vi "memory_stub.vi"() -> ()   [LabVIEW 2024, in "Nominal Client Engine.lvlib"]
uses:
  <vilib>/LabVIEW Open Source Project/Epoch Date & Time/formatter.iso8601/DateTime.ISO8601.lvclass
  <vilib>/LabVIEW Open Source Project/Epoch Date & Time/formatter.iso8601/ISO8601 Date Formats.ctl
  <vilib>/LabVIEW Open Source Project/Epoch Date & Time/formatter/DateTimeFormatter.lvclass
  <vilib>/LabVIEW Open Source Project/Epoch Date & Time/epoch.GPS/Epoch.GPS.lvclass
  <vilib>/LabVIEW Open Source Project/Epoch Date & Time/epoch/Epoch.lvclass
  <vilib>/LabVIEW Open Source Project/Epoch Date & Time/epoch.UNIX/Epoch.UNIX.lvclass
  <vilib>/LabVIEW Open Source Project/Epoch Date & Time/epoch.UTC/Epoch.UTC.lvclass
  <vilib>/LabVIEW Open Source Project/Epoch Date & Time/Epochs -- enum.ctl
  <vilib>/LabVIEW Open Source Project/Epoch Date & Time/UTC Offsets -- enum.ctl
  <vilib>/Nominal/Nominal IO Client/Nominal Client MultiPart Upload/Multipart Upload.lvclass
  <vilib>/Nominal/Nominal IO Client/Nominal Client/Nominal Client.lvclass
  <vilib>/addons/_JKI.lib/REST Client/classes/REST Client/REST Client.lvclass
  <vilib>/Utility/lvfile.llb/FT_FileTypes.ctl
  <vilib>/picture/picture.llb/imagedata.ctl
  <vilib>/addons/_JKI.lib/REST Client/classes/Response Headers/Response Headers.lvclass
  <vilib>/addons/_JKI.lib/REST Client/classes/REST Client/HTTP Header.ctl
  <vilib>/NI/Advanced HTTP Client/Header--Combo Box.ctl
  <vilib>/httpClient/MultipartData.ctl
  <vilib>/Nominal/Nominal IO Client/Run/Run.lvclass
  <vilib>/Nominal/Nominal IO Client/Run/Run Data.ctl
  <vilib>/LabVIEW Open Source Project/Epoch Date & Time/formatter.iso8601/ISO Day -- enum.ctl
  <vilib>/Nominal/Nominal IO Client/timestampMetadata/timestampMetadata.lvclass
  <vilib>/Utility/error.llb/whitespace.ctl
  <vilib>/Nominal/Nominal IO Client/ts.epochOfTimeUnit/ts.epochOfTimeUnit.lvclass
  <vilib>/Nominal/Nominal IO Client/ts.iso8601/ts.iso8601.lvclass
  <vilib>/Nominal/Nominal IO Client/ts.relative/ts.relative.lvclass
  Engine/Nominal Client Engine.lvlib
  <userlib>/_OpenG.lib/array/array.llb/openg_array.lvlib
  <userlib>/_OpenG.lib/array/array.llb/Conditional Auto-Indexing Tunnel (DBL)__ogtk.vi
  <userlib>/_OpenG.lib/array/array.llb/Delete Elements from 1D Array (DBL)__ogtk.vi
  <userlib>/_OpenG.lib/array/array.llb/Empty 1D Array (DBL)__ogtk.vi
  <userlib>/_OpenG.lib/array/array.llb/Filter 1D Array (DBL)__ogtk.vi
  <userlib>/_OpenG.lib/array/array.llb/Index 1D Array Elements (DBL)__ogtk.vi
  <userlib>/_OpenG.lib/array/array.llb/Remove Duplicates from 1D Array (DBL)__ogtk.vi
  <userlib>/_OpenG.lib/array/array.llb/Reorder 1D Array2 (DBL)__ogtk.vi
  <userlib>/_OpenG.lib/array/array.llb/Reorder 1D Array (DBL)__ogtk.vi
  <userlib>/_OpenG.lib/array/array.llb/Reverse 2D Array (Variant)__ogtk.vi
  <userlib>/_OpenG.lib/array/array.llb/Search 1D Array (DBL)__ogtk.vi
  <userlib>/_OpenG.lib/array/array.llb/Slice 1D Array (DBL)__ogtk.vi
  <userlib>/_OpenG.lib/array/array.llb/Sort 2D Array (DBL)__ogtk.vi
  <userlib>/_OpenG.lib/array/array.llb/Sort 1D Array (DBL)__ogtk.vi
  <vilib>/JDP Science/JDP Science Common Utilities/Base64/Base64 Support.lvlib
  <vilib>/Utility/Data Type/NI_Data Type.lvlib
  <vilib>/Utility/lvfile.llb/NI_FileType.lvlib
  <vilib>/Utility/LVLibp/NI_PackedLibraryUtility.lvlib
  <vilib>/NI/Advanced HTTP Client/Session.lvclass
  <vilib>/httpClient/LabVIEWHTTPClient.lvlib
panel:
  in  "prompt":string
  in  "error in":errorcluster
  in  "append to file? (new file:F)":bool
  in  "spreadsheet string":string
  in  "file path (dialog if empty)":path
  out "error out":errorcluster
  out "path":path
  in  "file path (dialog if empty) 2":path
  in  "format (%.3f)":string="%.3f"
  in  "2D data":dbl[][](array[numeric])
  in  "1D data":dbl[](array[numeric])
  in  "append to file? (new file:F) 2":bool
  in  "error in (no error)":errorcluster
  in  "transpose? (no:F)":bool
  in  "delimiter (\\t)":string="\t"
  out "new file path (Not A Path if cancelled)":path
  out "error out 2":errorcluster
  in  "file path (dialog if empty) 3":path
  in  "format (%s)":string="%s"
  in  "2D data 2":string[][](array[string])
  in  "1D data 2":string[](array[string])
  in  "append to file? (new file:F) 3":bool
  in  "error in (no error) 2":errorcluster
  in  "transpose? (no:F) 2":bool
  in  "delimiter (\\t) 2":string="\t"
  out "new file path (Not A Path if cancelled) 2":path
  out "error out 3":errorcluster
  in  "file path (dialog if empty) 4":path
  in  "format (%d)":string="%d"
  in  "2D data 3":i64[][](array[numeric])
  in  "1D data 3":i64[](array[numeric])
  in  "append to file? (new file:F) 4":bool
  in  "error in (no error) 3":errorcluster
  in  "transpose? (no:F) 3":bool
  in  "delimiter (\\t) 3":string="\t"
  out "new file path (Not A Path if cancelled) 3":path
  out "error out 4":errorcluster
  in  "file path (dialog if empty) 5":path
  in  "format (%.3f) 2":string="%.3f"
  in  "2D data 4":dbl[][](array[numeric])
  in  "1D data 4":dbl[](array[numeric])
  in  "append to file? (new file:F) 5":bool
  in  "error in (no error) 4":errorcluster
  in  "transpose? (no:F) 4":bool
  in  "delimiter (\\t) 4":string="\t"
  out "new file path (Not A Path if cancelled) 4":path
  out "error out 5":errorcluster
  in  "UTC Offset String":string
  out "Valid?":bool
  out "Offset (s)":ext
  out "UTC Offset":T1=enum."UTC+00:00"
  out "UTC Offset?":bool
  in  "error in 2":errorcluster
  in  "ts.relative in":refnum<class "ts.relative.lvclass">
  out "error out 6":errorcluster
  out "JSON Object":string
  out "ts.relative out":refnum<class "ts.relative.lvclass">
  in  "Time Unit":T2(ring)
  in  "Time Series Name":string
  out "ts.relative out 2":refnum<class "ts.relative.lvclass">
  in  "error in 3":errorcluster
  in  "ts.iso8601 in":refnum<class "ts.iso8601.lvclass">
  out "error out 7":errorcluster
  out "JSON Object 2":string
  out "ts.iso8601 out":refnum<class "ts.iso8601.lvclass">
  in  "Time Series Name 2":string
  out "ts.iso8601 out 2":refnum<class "ts.iso8601.lvclass">
  in  "error in 4":errorcluster
  in  "ts.epochOfTimeUnit in":refnum<class "ts.epochOfTimeUnit.lvclass">
  out "error out 8":errorcluster
  out "JSON Object 3":string
  out "ts.epochOfTimeUnit out":refnum<class "ts.epochOfTimeUnit.lvclass">
  in  "Time Unit 2":T2(ring)
  in  "Time Series Name 3":string
  out "ts.epochOfTimeUnit out 2":refnum<class "ts.epochOfTimeUnit.lvclass">
  in  "string":string
  in  "location (both)":T3 items=["both", "start of string", "end of string"]
  out "trimmed string":string
  in  "string 2":string
  in  "reverse?":bool
  in  "enable?":bool
  out "trimmed string 2":string
  out "timestampMetadata out":refnum<class "timestampMetadata.lvclass">
  in  "error in 5":errorcluster
  in  "Object To Update":string
  in  "JSON in":string
  in  "timestampMetadata in":refnum<class "timestampMetadata.lvclass">
  out "error out 9":errorcluster
  out "JSON out":string
  out "timestampMetadata out 2":refnum<class "timestampMetadata.lvclass">
  in  "error in 6":errorcluster
  in  "Object Name":string="timestampMetadata"
  in  "JSON in 2":string
  in  "timestampMetadata in 2":refnum<class "timestampMetadata.lvclass">
  out "error out 10":errorcluster
  out "JSON out 2":string
  out "timestampMetadata out 3":refnum<class "timestampMetadata.lvclass">
  in  "error in 7":errorcluster
  in  "timestampMetadata in 3":refnum<class "timestampMetadata.lvclass">
  out "error out 11":errorcluster
  out "JSON Object 4":string
  out "timestampMetadata out 4":refnum<class "timestampMetadata.lvclass">
  out "timestampMetadata out 5":refnum<class "timestampMetadata.lvclass">
  in  "UTC? (F)":bool
  in  "Timestamp (now)":timestamp
  out "is Leap Year?":bool
  out "year":i32
  in  "UTC? (F) 2":bool
  in  "Timestamp (now) 2":timestamp
  out "ISO8601 Ordinal Date":string
  out "ISO8601 Weekday":string
  out "ISO8601 Week":string
  in  "UTC? (F) 3":bool
  in  "Timestamp (now) 3":timestamp
  out "ISO8601 UTC DateTime":string
  in  "UTC? (F) 4":bool
  in  "Timestamp (now) 4":timestamp
  out "Day of Year":i32
  out "ISO Weekday":i32
  out "ISO Day":T4
  in  "UTC? (F) 5":bool
  in  "Timestamp (now) 5":timestamp
  out "ISO8601 Calendar Month":string
  out "ISO8601 Date":string
  out "String":string
  in  "Run Data":T5
  out "Run":refnum<class "Run.lvclass">
  in  "error in (no error) 5":errorcluster
  in  "REST Client in":refnum<class "REST Client.lvclass">
  out "error out 12":errorcluster
  in  "request specific headers":T6[](array[typedef])
  in  "timeout (0 = Use Default)":i32
  in  "error in (no error) 6":errorcluster
  in  "Request body":string
  in  "Path":string
  in  "REST Client in 2":refnum<class "REST Client.lvclass">
  out "error out 13":errorcluster
  out "Response body":string
  out "Response Headers":refnum<class "Response Headers.lvclass">
  out "REST Client out":refnum<class "REST Client.lvclass">
  out "Status String":string
  out "Status Code":u16
  in  "request specific headers 2":T6[](array[typedef])
  in  "timeout (0 = Use Default) 2":i32
  in  "error in (no error) 7":errorcluster
  in  "Path 2":string
  in  "REST Client in 3":refnum<class "REST Client.lvclass">
  out "error out 14":errorcluster
  out "Response body 2":string
  out "Response Headers 2":refnum<class "Response Headers.lvclass">
  out "REST Client out 2":refnum<class "REST Client.lvclass">
  out "Status String 2":string
  out "Status Code 2":u16
  in  "request specific headers 3":T6[](array[typedef])
  in  "timeout (0 = Use Default) 3":i32
  in  "error in (no error) 8":errorcluster
  in  "Multipart Post data":T8[](array[typedef])
  in  "Path 3":string
  in  "REST Client in 4":refnum<class "REST Client.lvclass">
  out "error out 15":errorcluster
  out "Response body 3":string
  out "Response Headers 3":refnum<class "Response Headers.lvclass">
  out "REST Client out 3":refnum<class "REST Client.lvclass">
  out "Status String 3":string
  out "Status Code 3":u16
  in  "request specific headers 4":T6[](array[typedef])
  in  "timeout (0 = Use Default) 4":i32
  in  "error in (no error) 9":errorcluster
  in  "Request body 2":string
  in  "Path 4":string
  in  "REST Client in 5":refnum<class "REST Client.lvclass">
  out "error out 16":errorcluster
  out "Response body 4":string
  out "Response Headers 4":refnum<class "Response Headers.lvclass">
  out "REST Client out 4":refnum<class "REST Client.lvclass">
  out "Status String 4":string
  out "Status Code 4":u16
  in  "request specific headers 5":T6[](array[typedef])
  in  "timeout (0 = Use Default) 5":i32
  in  "error in (no error) 10":errorcluster
  in  "Request body 3":string
  in  "Path 5":string
  in  "REST Client in 6":refnum<class "REST Client.lvclass">
  out "error out 17":errorcluster
  out "Response body 5":string
  out "Response Headers 5":refnum<class "Response Headers.lvclass">
  out "REST Client out 5":refnum<class "REST Client.lvclass">
  out "Status String 5":string
  out "Status Code 5":u16
  in  "request specific headers 6":T6[](array[typedef])
  in  "timeout (0 = Use Default) 6":i32
  in  "error in (no error) 11":errorcluster
  in  "Path 6":string
  in  "REST Client in 7":refnum<class "REST Client.lvclass">
  out "error out 18":errorcluster
  out "Response body 6":string
  out "Response Headers 6":refnum<class "Response Headers.lvclass">
  out "REST Client out 6":refnum<class "REST Client.lvclass">
  out "Status String 6":string
  out "Status Code 6":u16
  in  "request specific headers 7":T6[](array[typedef])
  in  "timeout (0 = Use Default) 7":i32
  in  "error in (no error) 12":errorcluster
  in  "Path 7":string
  in  "REST Client in 8":refnum<class "REST Client.lvclass">
  out "error out 19":errorcluster
  out "Response body 7":string
  out "Response Headers 7":refnum<class "Response Headers.lvclass">
  out "REST Client out 7":refnum<class "REST Client.lvclass">
  out "Status String 7":string
  out "Status Code 7":u16
  in  "Default Headers ([JSON])":T6[](array[typedef])=[{"header"="Content-Type", "value"="application/json"}]
  in  "REST Client in 9":refnum<class "REST Client.lvclass">
  in  "Verify Server(true)":bool=TRUE
  in  "Cookie File":path
  in  "error in (no error) 13":errorcluster
  in  "Authentication":cluster{"Username":string, "Password":string}
  in  "Escape URLs (true)":bool=TRUE
  in  "Base URL":string
  out "error out 20":errorcluster
  out "REST Client out 8":refnum<class "REST Client.lvclass">
  in  "error in (no error) 14":errorcluster
  in  "Response Headers in":refnum<class "Response Headers.lvclass">
  out "error out 21":errorcluster
  out "Values":string[](array[string])
  out "Names":string[](array[string])
  out "Response Headers out":refnum<class "Response Headers.lvclass">
  in  "error in (no error) 15":errorcluster
  in  "Name":string
  in  "Response Headers in 2":refnum<class "Response Headers.lvclass">
  out "error out 22":errorcluster
  out "Found?":bool
  out "Value":string
  out "Response Headers out 2":refnum<class "Response Headers.lvclass">
  in  "error in (no error) 16":errorcluster
  in  "vi reference":refnum<vi>
  out "error out 25":errorcluster
  out "packed library path":path
  out "vi reference out":refnum<vi>
  in  "error in (no error) 17":errorcluster
  in  "packed library path 2":path
  out "error out 26":errorcluster
  out "source project path":path
  in  "error in (no error) 18":errorcluster
  in  "packed library path 3":path
  out "error out 27":errorcluster
  out "guid":string
  in  "error in (no error) 19":errorcluster
  in  "qualified name":string
  in  "packed library path 4":path
  out "error out 28":errorcluster
  out "path 2":path
  in  "error in (no error) 20":errorcluster
  in  "packed library path 5":path
  out "error out 29":errorcluster
  out "paths":path[](array[path])
  out "qualified names":string[](array[string])
  in  "error in (no error) 21":errorcluster
  in  "Enable":bool
  out "error out 30":errorcluster
  in  "file type":T9
  out "Is LabVIEW document?":bool
  in  "file type 2":T9
  out "Is library type?":bool
  in  "file type 3":T9
  out "Can be in LLB?":bool
  in  "error in (no error) 22":errorcluster
  in  "is template?":bool
  in  "file type 4":T9
  out "error out 31":errorcluster
  out "image data":T10
  in  "file type 5":T9
  out "Is VI?":bool
  in  "error in (no error) 23":errorcluster
  in  "path 3":path
  out "error out 32":errorcluster
  out "Is LLB?":bool
  in  "error in (no error) 24":errorcluster
  in  "path 4":path
  out "error out 33":errorcluster
  out "Is Class Private Data Control?":bool
  out "Is VI? 2":bool
  in  "error in (no error) 25":errorcluster
  in  "path 5":path
  out "error out 34":errorcluster
  out "Is library type? 2":bool
  in  "error in (no error) 26":errorcluster
  in  "path 6":path
  out "error out 35":errorcluster
  out "Is LabVIEW document? 2":bool
  in  "error in (no error) 27":errorcluster
  in  "path 7":path
  out "error out 36":errorcluster
  out "image data 2":T10
  in  "error in (no error) 28":errorcluster
  in  "path 8":path
  out "error out 37":errorcluster
  out "is template? 2":bool
  out "file type 6":T9
  in  "error in (no error) 29":errorcluster
  in  "path 9":path
  out "error out 38":errorcluster
  out "Can be in LLB? 2":bool
  in  "error in (no error) 30":errorcluster
  in  "variant":variant
  out "error out 39":errorcluster
  out "default palette path":path
  in  "error in 10":errorcluster
  in  "Multipart Upload in":refnum<class "Multipart Upload.lvclass">
  out "error out 40":errorcluster
  out "Multipart Upload out":refnum<class "Multipart Upload.lvclass">
  in  "Part Number":i32
  in  "error in 11":errorcluster
  in  "File Part Binary":string
  in  "Multipart Upload":refnum<class "Multipart Upload.lvclass">
  out "error out 41":errorcluster
  out "Multipart Upload out 2":refnum<class "Multipart Upload.lvclass">
  in  "Part Number 2":i32
  in  "error in 12":errorcluster
  in  "Multipart Upload in 2":refnum<class "Multipart Upload.lvclass">
  out "error out 42":errorcluster
  out "Multipart Upload out 3":refnum<class "Multipart Upload.lvclass">
  in  "error in 13":errorcluster
  in  "Body":string
  in  "Full Path":string
  in  "REST Client":refnum<class "REST Client.lvclass">
  out "error out 43":errorcluster
  out "Response":string
  in  "error in 14":errorcluster
  in  "Multipart Upload 2":refnum<class "Multipart Upload.lvclass">
  out "error out 44":errorcluster
  out "Multipart Upload out 4":refnum<class "Multipart Upload.lvclass">
  in  "error in 15":errorcluster
  in  "File Path":path
  in  "Nominal Client in":refnum<class "Nominal Client.lvclass">
  out "error out 45":errorcluster
  out "Multipart Upload 3":refnum<class "Multipart Upload.lvclass">
  out "Nominal Client out":refnum<class "Nominal Client.lvclass">
  in  "error in 16":errorcluster
  in  "Multipart Upload in 3":refnum<class "Multipart Upload.lvclass">
  out "error out 46":errorcluster
  out "S3 Path to File":string
  in  "error in 17":errorcluster
  in  "Multipart Upload 4":refnum<class "Multipart Upload.lvclass">
  out "error out 47":errorcluster
  in  "error in 18":errorcluster
  in  "MultiPart Upload":refnum<class "Multipart Upload.lvclass">
  out "error out 48":errorcluster
  in  "error in 19":errorcluster
  in  "Key":string
  in  "Upload ID":string
  out "error out 49":errorcluster
  out "Nominal Client MultiPart Upload":refnum<class "Multipart Upload.lvclass">
  in  "Adjust for Local DST? (T)":bool=TRUE
  in  "Strict ISO? (T)":bool=TRUE
  in  "ISO8601 Date String":string
  out "valid?":bool
  out "ISO Format":T11
  out "Timestamp":timestamp
  in  "timestamp (now)":timestamp
  out "is Leap Year? 2":bool
  in  "Year (0: this year)":i32
  out "is Leap Year? 3":bool
  in  "timestamp (now) 2":timestamp
  out "is DST?":bool
  in  "path 10":path
  out "Is Path and Not Empty?":bool
  in  "Year (0: this year) 2":i32
  out "Month Lengths":i32[](array[numeric])
  in  "error in (no error) 31":errorcluster
  in  "object":refnum<class>
  out "error out 50":errorcluster
  out "class name":string
  in  "UTC? (F) 6":bool
  out "UTC Offset String 2":string
  out "UTC Offset 2":T1=enum."UTC+00:00"
  in  "error in (no error) 32":errorcluster
  in  "file":path
  out "error out 51":errorcluster
  out "filename without extension":string
  out "lowercase file extension":string
  out "dup file":path
  out "unmodified file extension":string
  in  "Timestamp (now) 6":timestamp
  in  "Epoch (Local)":refnum<class "Epoch.lvclass">
  out "Fractional Second":dbl format="%#.19f"
  out "Epoch Time (s)":i64
  out "Epoch out":refnum<class "Epoch.lvclass">
  in  "is warning? (False)":bool
  in  "show call chain? (False)":bool
  in  "error in (no error) 33":errorcluster
  in  "error message (\"\")":string
  in  "error code (0)":i32
  out "error out 52":errorcluster
  in  "Epoch (UTC)":T12=enum."UTC"
  in  "Epoch Time":ext format="%#.6f"
  out "Not a Timestamp?":bool
  in  "Use TAI Offset?":bool
  in  "Fractional Second 2":dbl format="%#.6f"
  in  "UTC Time (s)":i64
  in  "Epoch (UTC) 2":refnum<class "Epoch.UTC.lvclass">
  out "Not a Timestamp? 2":bool
  out "Timestamp 2":timestamp
  out "Epoch out 2":refnum<class "Epoch.UTC.lvclass">
  in  "Epoch":refnum<class "Epoch.UTC.lvclass">
  out "Offset to UTC":i64
  in  "Use TAI Offset? 2":bool
  in  "Fractional Second 3":dbl format="%#.6f"
  in  "Unix Time (s)":i64
  in  "Epoch (Unix)":refnum<class "Epoch.UNIX.lvclass">
  out "Not a Timestamp? 3":bool
  out "Timestamp 3":timestamp
  out "Epoch out 3":refnum<class "Epoch.UNIX.lvclass">
  in  "Epoch (UNIX)":refnum<class "Epoch.UNIX.lvclass">
  out "Offset to UTC 2":i64
  in  "(Integer) Time (us)":i64
  in  "Epoch in":refnum<class "Epoch.lvclass">
  out "Fractional Second 4":dbl format="%#.6f"
  out "(Integer) Time (s)":i64
  out "Epoch out 4":refnum<class "Epoch.lvclass">
  in  "(Integer) Time (ms)":i64
  in  "Epoch in 2":refnum<class "Epoch.lvclass">
  out "Fractional Second 5":dbl format="%#.6f"
  out "(Integer) Time (s) 2":i64
  out "Epoch out 5":refnum<class "Epoch.lvclass">
  in  "(Float) Time (s)":dbl format="%#.6f"
  in  "Epoch in 3":refnum<class "Epoch.lvclass">
  out "Fractional Second 6":dbl format="%#.6f"
  out "(Integer) Time (s) 3":i64
  out "Epoch out 6":refnum<class "Epoch.lvclass">
  in  "Fractional Second 7":dbl format="%#.6f"
  in  "(Integer) Time (s) 4":i64
  in  "Epoch in 4":refnum<class "Epoch.lvclass">
  out "(Integer) Time (us) 2":i64
  out "Epoch out 7":refnum<class "Epoch.lvclass">
  in  "Fractional Second 8":dbl format="%#.6f"
  in  "(Integer) Time (s) 5":i64
  in  "Epoch in 5":refnum<class "Epoch.lvclass">
  out "(Integer) Time (ms) 2":i64
  out "Epoch out 8":refnum<class "Epoch.lvclass">
  in  "Fractional Second 9":dbl format="%#.6f"
  in  "(Integer) Time (s) 6":i64
  in  "Epoch in 6":refnum<class "Epoch.lvclass">
  out "(Float) Time (s) 2":dbl format="%#.6f"
  out "Epoch out 9":refnum<class "Epoch.lvclass">
  in  "UTC Epoch Time":i64=2272060800
  out "Leap Seconds":i64=2272060800
  out "Leap Seconds 2":i64[](array[numeric])
  out "UTC Time":i64[](array[numeric])
  in  "DateTimeFormatter (ISO8601)":refnum<class "DateTimeFormatter.lvclass">
  in  "UTC? (F) 7":bool
  in  "Fractional Second 10":dbl format="%#.6f"
  in  "Epoch Time (s) 2":i64
  in  "Epoch 2":refnum<class "Epoch.lvclass">
  out "Not a Timestamp? 4":bool
  out "DateTime string":string
  out "Epoch out 10":refnum<class "Epoch.lvclass">
  in  "Use TAI Offset? 3":bool
  in  "Fractional Second 11":dbl format="%#.6f"
  in  "Epoch Time (s) 3":i64
  in  "Epoch (Local) 2":refnum<class "Epoch.lvclass">
  out "Not a Timestamp? 5":bool
  out "Timestamp 4":timestamp
  out "Epoch (out)":refnum<class "Epoch.lvclass">
  in  "Reference Time":timestamp
  out "Timestamp Offset":i64
  in  "Epoch Time 2":i64=2272060800
  in  "Epoch 3":refnum<class "Epoch.lvclass">
  out "Offset to TAI":i64
  in  "Epoch 4":refnum<class "Epoch.lvclass">
  out "Offset to UTC 3":i64
  in  "Use TAI Offset? 4":bool=TRUE
  in  "Fractional Second 12":dbl format="%#.6f"
  in  "GPS Time (s)":i64
  in  "Epoch (GPS)":refnum<class "Epoch.GPS.lvclass">
  out "Not a Timestamp? 6":bool
  out "Timestamp 5":timestamp
  out "Epoch out 11":refnum<class "Epoch.GPS.lvclass">
  in  "Epoch (GPS) 2":refnum<class "Epoch.GPS.lvclass">
  out "Offset to UTC 4":i64
  in  "Epoch Time 3":i64=2272060800
  in  "Epoch.GPS":refnum<class "Epoch.GPS.lvclass">
  out "Offset to TAI 2":i64
  in  "DateTime String":string
  in  "DateTimeFormatter in":refnum<class "DateTimeFormatter.lvclass">
  out "Timestamp 6":timestamp
  out "DateTimeFormatter out":refnum<class "DateTimeFormatter.lvclass">
  in  "UTC? (F) 8":bool
  in  "Timestamp (now) 7":timestamp
  in  "DateTimeFormatter in 2":refnum<class "DateTimeFormatter.lvclass">
  out "DateTime String 2":string
  out "DateTimeFormatter out 2":refnum<class "DateTimeFormatter.lvclass">
  in  "DateTime String 3":string
  in  "DateTimeFormatter in 3":refnum<class "DateTimeFormatter.lvclass">
  out "Not a Timestamp? 7":bool
  out "Timestamp 7":timestamp
  out "DateTimeFormatter out 3":refnum<class "DateTimeFormatter.lvclass">
  in  "UTC? (F) 9":bool
  in  "Timestamp (now) 8":timestamp
  in  "DateTimeFormatter in 4":refnum<class "DateTimeFormatter.lvclass">
  out "Not a Timestamp? 8":bool
  out "DateTime String 4":string
  out "DateTimeFormatter out 4":refnum<class "DateTimeFormatter.lvclass">
  in  "Adjust for DST? (T)":bool=TRUE
  in  "Timestamp 8":timestamp
  out "Adjusted Timestamp":timestamp
  in  "year 2":i32
  out "First Day of W01":timestamp
  in  "DateTime String 5":string
  in  "DateTime.ISO8601 in":refnum<class "DateTime.ISO8601.lvclass">
  out "Timestamp 9":timestamp
  out "DateTime.ISO8601 out":refnum<class "DateTime.ISO8601.lvclass">
  in  "UTC? (F) 10":bool
  in  "Timestamp (now) 9":timestamp
  in  "DateTime.ISO8601 in 2":refnum<class "DateTime.ISO8601.lvclass">
  out "DateTime String 6":string
  out "DateTime.ISO8601 out 2":refnum<class "DateTime.ISO8601.lvclass">
  in  "Support RFC3339 (T)":bool=TRUE
  in  "DateTime.ISO8601 in 3":refnum<class "DateTime.ISO8601.lvclass">
  out "DateTime.ISO8601 out 3":refnum<class "DateTime.ISO8601.lvclass">
  in  "DateTime.ISO8601 in 4":refnum<class "DateTime.ISO8601.lvclass">
  out "Support RFC3339":bool=TRUE
  out "DateTime.ISO8601 out 4":refnum<class "DateTime.ISO8601.lvclass">
  in  "ISO Format 2":T11
  in  "DateTime.ISO8601 in 5":refnum<class "DateTime.ISO8601.lvclass">
  out "DateTime.ISO8601 out 5":refnum<class "DateTime.ISO8601.lvclass">
  in  "DateTime.ISO8601 in 6":refnum<class "DateTime.ISO8601.lvclass">
  out "ISO Format 3":T11
  out "DateTime.ISO8601 out 6":refnum<class "DateTime.ISO8601.lvclass">
  in  "error in (no error) 34":errorcluster
  in  "specific error code to clear (0: all)":i32
  out "error out 53":errorcluster
  out "specific error cleared?":bool
  in  "error in (no error) 35":errorcluster
  in  "path 11":path
  out "error out 54":errorcluster
  out "file or folder exists?":bool
  out "dup path":path
  in  "Base64 or Base64URL":string
  out "Decoded":string
  in  "Padding (T)":bool=TRUE
  in  "String to Encode":string
  out "Base64 Encoded":string
  in  "Padding (F)":bool
  in  "String to Encode 2":string
  out "Base64URL Encoded":string
  out "Application Directory":path
  in  "Order":enum16{"ascending", "descending"}(ring)
  in  "Array in":dbl[](array[numeric]) format="%.2f"
  out "Sorted Pointers":i32[](array[numeric])
  out "Sorted Array out":dbl[](array[numeric]) format="%.2f"
  in  "Column/Row to Sort By":u32
  in  "Sort By in":enum16{"row", "column"}(ring)
  in  "Order 2":enum16{"ascending", "descending"}(ring)
  in  "Array in 2":dbl[][](array[numeric]) format="%.2f"
  out "Sort By out":enum16{"row", "column"}(ring)
  out "Index Out of Range?":bool
  out "Sorted Pointers 2":i32[](array[numeric])
  out "Sorted Array out 2":dbl[][](array[numeric]) format="%.2f"
  in  "slice":string caption="subset (i:j)"
  in  "array":dbl[](array[numeric]) format="%.2f"
  out "subarray (array[i:j])":dbl[](array[numeric]) format="%.2f"
  in  "Array":dbl[](array[numeric]) format="%.2f"
  in  "Element Data":dbl format="%.2f"
  in  "Start Index (0)":i32
  out "Indices of Elements":i32[](array[numeric])
  in  "by rows or columns (rows)":enum16{"rows", "columns"}(ring)
  in  "Array 2":variant[][](array[variant])
  out "Reversed Array":variant[][](array[variant])
  in  "Sorted Pointers in":i32[](array[numeric])
  in  "Array in 3":dbl[](array[numeric]) format="%.2f"
  out "Sorted Pointers out":i32[](array[numeric])
  out "Sorted Array out 3":dbl[](array[numeric]) format="%.2f"
  in  "indices":i32[](array[numeric])
  in  "array 2":dbl[](array[numeric]) format="%.2f"
  out "reordered array":dbl[](array[numeric]) format="%.2f"
  in  "Input Array":dbl[](array[numeric]) format="%.2f"
  out "Output Array":dbl[](array[numeric]) format="%.2f"
  out "indices of removed elements":i32[](array[numeric])
  in  "indices 2":i32[](array[numeric])
  in  "array 3":dbl[](array[numeric]) format="%.2f"
  out "elements":dbl[](array[numeric]) format="%.2f"
  in  "items to filter":dbl[](array[numeric]) format="%.2f"
  in  "array 4":dbl[](array[numeric]) format="%.2f"
  out "filtered item indices":i32[](array[numeric])
  out "filtered array":dbl[](array[numeric]) format="%.2f"
  in  "Array 3":dbl[](array[numeric]) format="%.2f"
  out "Empty Array?":bool
  in  "indices 3":i32[](array[numeric])
  in  "array 5":dbl[](array[numeric]) format="%.2f"
  out "deleted elements":dbl[](array[numeric]) format="%.2f"
  out "array w/ subset deleted":dbl[](array[numeric]) format="%.2f"
  in  "Array in 4":dbl[](array[numeric]) format="%.2f"
  in  "Elements to keep":bool[](array[boolean])
  out "Filtered Array out":dbl[](array[numeric]) format="%.2f"
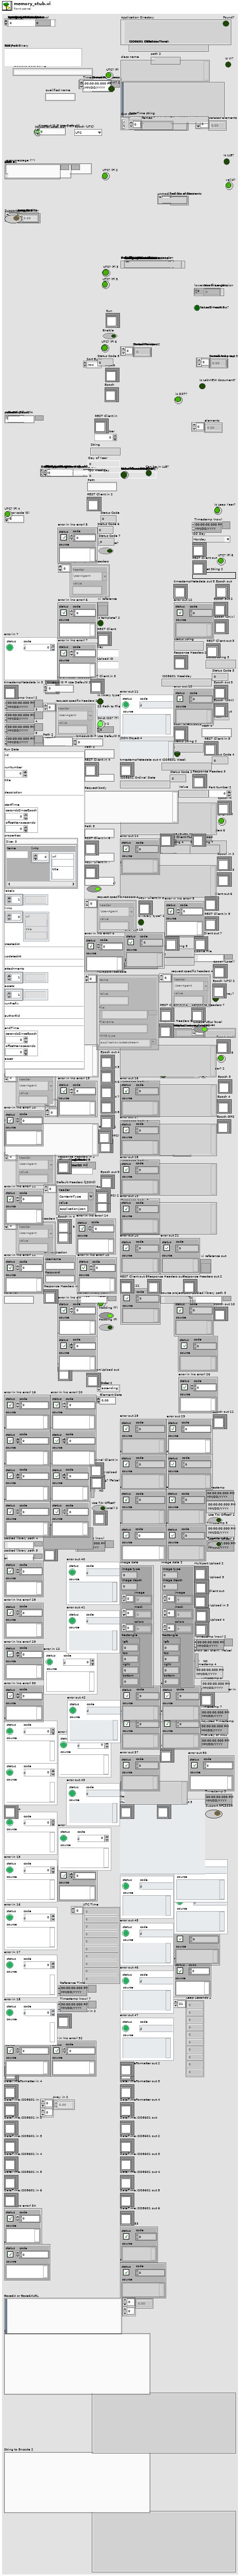
[diagram p1: front panel]
types:
  T1 = typedef "UTC Offsets -- enum.ctl" = enum16{"UTC-12:00", "UTC-11:00", "UTC-10:00", "UTC-09:30", "UTC-09:00", "UTC-08:00", "UTC-07:00", "UTC-06:00", "UTC-05:00", "UTC-04:00", "UTC-03:30", "UTC-03:00", "UTC-02:00", "UTC-01:00", "UTC-00:00", "UTC+00:00", "UTC+01:00", "UTC+02:00", "UTC+03:00", "UTC+03:30", "UTC+04:00", "UTC+04:30", "UTC+05:00", "UTC+05:30", "UTC+05:45", "UTC+06:00", "UTC+06:30", "UTC+07:00", "UTC+08:00", "UTC+08:45", "UTC+09:00", "UTC+09:30", "UTC+10:00", "UTC+10:30", "UTC+11:00", "UTC+12:00", "UTC+12:45", "UTC+13:00", "UTC+14:00"}
  T2 = enum16{"DAYS", "HOURS", "MINUTES", "SECONDS", "MILLISECONDS", "MICROSECONDS", "NANOSECONDS", "PICOSECONDS"}
  T3 = typedef "whitespace.ctl" = u16
  T4 = typedef "ISO Day -- enum.ctl" = enum16{"Monday", "Tuesday", "Wednesday", "Thursday", "Friday", "Saturday", "Sunday"}
  T5 = typedef "Run.lvclass/Run Data.ctl" = cluster{"rid":string, "runNumber":i32, "title":string, "description":string, "startTime":cluster{"secondsSinceEpoch":i32, "offsetNanoseconds":i32}, "properties":map{string, cluster{"url":string, "title":string}[]}, "labels":string[], "links":cluster{"url":string, "title":string}[], "createdAt":string, "updatedAt":string, "attachments":string[], "assets":string[], "runPrefix":string, "authorRid":string, "endTime":cluster{"secondsSinceEpoch":i32, "offsetNanoseconds":i32}, "asset":string}
  T6 = typedef "REST Client.lvlib/REST Client.lvclass/HTTP Header.ctl" = cluster{"header":T7, "value":string}
  T7 = typedef "lib_NI_Advanced HTTP Client.lvlib/Session.lvclass/Header--Combo Box.ctl" = string
  T8 = typedef "LabVIEWHTTPClient.lvlib/MultipartData.ctl" = cluster{"Name":string, "Value":string, "File":path, "Filename":string, "MIME type":string}
  T9 = typedef "NI_FileType.lvlib/FT_FileTypes.ctl" = enum32{"Invalid file/path", "Unknown type", "Instrument", "Control", "Polymorphic VI", "Project", "Library", "LVClass", "XControl", "XNode", "CIN", "Run-time menu", "Palette menu", "LLB", "Shortcut", "Directory", "Class Private Data Control", "Statechart", "MathScript .m file", "Ladder Diagram", "LVLibp"}
  T10 = typedef "imagedata.ctl" = cluster{"image type":i32, "image depth":i32, "image":u8[], "mask":u8[], "colors":u32[], "Rectangle":cluster{"left":i16, "top":i16, "right":i16, "bottom":i16}}
  T11 = typedef "ISO8601 Date Formats.ctl" = enum16{"UTC Date-Time", "Date", "Calendar Month", "Week", "Week-Day", "Month-Day", "Ordinal Date"}
  T12 = typedef "Epochs -- enum.ctl" = enum16{"Local", "UTC", "Unix", "GPS"}
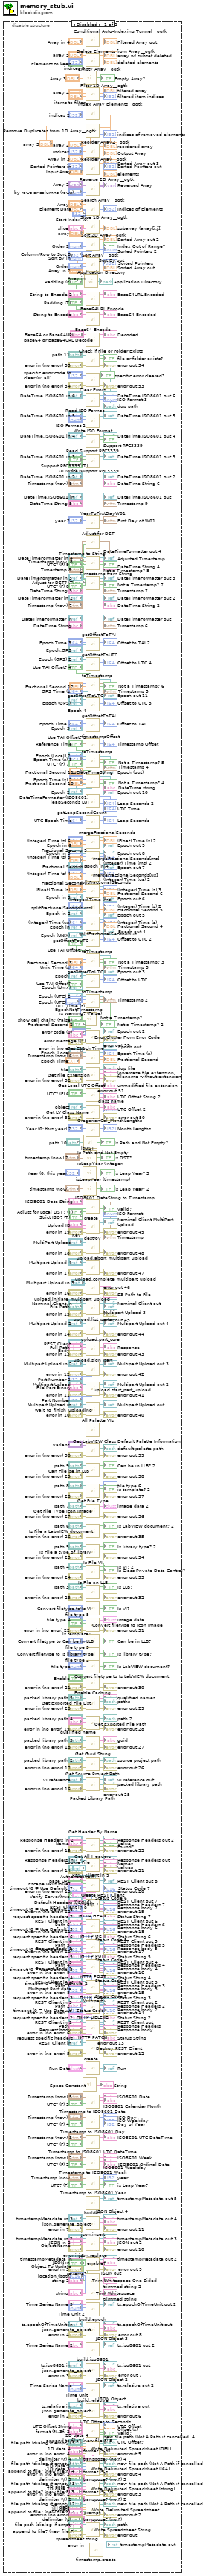
[diagram p0: block diagram]
diagram:
  n1 = disable-structure shown="Disabled" {
    frame Disabled {
      n2 = call <vilib>:"Space Constant.vi"() -> ("String"=→"String":string)
      n3 = call-poly <userlib>:"Empty Array__ogtk.vi"("Array"="Array 3") -> ("Empty Array?"=→"Empty Array?":bool)  [unwired: 8 in]
      n4 = call <vilib>:"EpochNotTimestamp.vi"("Epoch (UTC)"="Epoch (UTC)", "Epoch Time"="Epoch Time") -> ("Not a Timestamp?"=→"Not a Timestamp?":bool)  [unwired: 7 in]
      n5 = call <vilib>:"isDST.vi"("timestamp (now)"="timestamp (now) 2") -> ("is DST?"=→"is DST?":bool)  [unwired: 8 in]
      n6 = call <vilib>:"isLeapYear (integer).vi"("Year (0: this year)"="Year (0: this year)") -> ("is Leap Year?"=→"is Leap Year? 3":bool)  [unwired: 8 in]
      n7 = call <vilib>:"isLeapYear (timestamp).vi"("timestamp (now)"="timestamp (now)") -> ("is Leap Year?"=→"is Leap Year? 2":bool)  [unwired: 8 in]
      n8 = call <vilib>:"Is Path and Not Empty.vi"("path"="path 10") -> ("Is Path and Not Empty?"=→"Is Path and Not Empty?":bool)  [unwired: 4 in]
      n9 = call <vilib>:"Application Directory.vi"() -> ("Application Directory"=→"Application Directory":path)
      n10 = call-poly <userlib>:"Conditional Auto-Indexing Tunnel__ogtk.vi"("Array in"="Array in 4", "Elements to keep"="Elements to keep") -> ("Filtered Array out"=→"Filtered Array out":dbl[])  [unwired: 5 in]
      n11 = call-poly <userlib>:"Delete Elements from Array__ogtk.vi"("indices"="indices 3", "array"="array 5") -> ("deleted elements"=→"deleted elements":dbl[], "array w/ subset deleted"=→"array w/ subset deleted":dbl[])  [unwired: 8 in]
      n12 = call-poly <userlib>:"Filter 1D Array__ogtk.vi"("items to filter"="items to filter", "array"="array 4") -> ("filtered item indices"=→"filtered item indices":i32[], "filtered array"=→"filtered array":dbl[])  [unwired: 4 in]
      n13 = call-poly <userlib>:"Index Array Elements__ogtk.vi"("indices"="indices 2", "array"="array 3") -> ("elements"=→"elements":dbl[])  [unwired: 9 in]
      n14 = call-poly <userlib>:"Remove Duplicates from 1D Array__ogtk.vi"("Input Array"="Input Array") -> ("Output Array"=→"Output Array":dbl[], "indices of removed elements"=→"indices of removed elements":i32[])
      n15 = call-poly <userlib>:"Reorder Array2__ogtk.vi"("indices"="indices", "array"="array 2") -> ("reordered array"=→"reordered array":dbl[])  [unwired: 9 in]
      n16 = call-poly <userlib>:"Reorder Array__ogtk.vi"("Sorted Pointers in"="Sorted Pointers in", "Array in"="Array in 3") -> ("Sorted Pointers out"=→"Sorted Pointers out":i32[], "Sorted Array out"=→"Sorted Array out 3":dbl[])  [unwired: 8 in]
      n17 = call-poly <userlib>:"Reverse 2D Array__ogtk.vi"("by rows or columns (rows)"="by rows or columns (rows)", "Array"="Array 2") -> ("Reversed Array"=→"Reversed Array":variant[][])  [unwired: 1 in]
      n18 = call-poly <userlib>:"Search Array__ogtk.vi"("Array"="Array", "Element Data"="Element Data", "Start Index (0)"="Start Index (0)") -> ("Indices of Elements"=→"Indices of Elements":i32[])  [unwired: 6 in]
      n19 = call-poly <userlib>:"Slice 1D Array__ogtk.vi"("slice"="slice", "array"="array") -> ("subarray (array[i:j])"=→"subarray (array[i:j])":dbl[])  [unwired: 5 in]
      n20 = call-poly <userlib>:"Sort 2D Array__ogtk.vi"("Column/Row to Sort By"="Column/Row to Sort By", "Sort By in"="Sort By in", "Order"="Order 2", "Array in"="Array in 2") -> ("Sort By out"=→"Sort By out":enum16{"row", "column"}, "Index Out of Range?"=→"Index Out of Range?":bool, "Sorted Pointers"=→"Sorted Pointers 2":i32[], "Sorted Array out"=→"Sorted Array out 2":dbl[][])  [unwired: 4 in]
      n21 = call-poly <userlib>:"Sort Array__ogtk.vi"("Order"="Order", "Array in"="Array in") -> ("Sorted Pointers"=→"Sorted Pointers":i32[], "Sorted Array out"=→"Sorted Array out":dbl[])  [unwired: 8 in]
      n22 = call <vilib>:"Base64URL Encode.vi"("Padding (F)"="Padding (F)", "String to Encode"="String to Encode 2") -> ("Base64URL Encoded"=→"Base64URL Encoded":string)  [unwired: 9 in]
      n23 = call <vilib>:"Base64 Encode.vi"("Padding (T)"="Padding (T)", "String to Encode"="String to Encode") -> ("Base64 Encoded"=→"Base64 Encoded":string)  [unwired: 9 in]
      n24 = call <vilib>:"Base64 or Base64URL Decode.vi"("Base64 or Base64URL"="Base64 or Base64URL") -> ("Decoded"=→"Decoded":string)  [unwired: 10 in]
      n25 = call <vilib>:"Check if File or Folder Exists.vi"("error in (no error)"="error in (no error) 35", "path"="path 11") -> ("error out"=→"error out 54":errorcluster, "file or folder exists?"=→"file or folder exists?":bool, "dup path"=→"dup path":path)  [unwired: 7 in]
      n26 = call <vilib>:"Clear Errors.vi"("error in (no error)"="error in (no error) 34", "specific error code to clear (0: all)"="specific error code to clear (0: all)") -> ("error out"=→"error out 53":errorcluster, "specific error cleared?"=→"specific error cleared?":bool)  [unwired: 4 in]
      n27 = call <vilib>:"Read ISO Format.vi"("DateTime.ISO8601 in"="DateTime.ISO8601 in 6") -> ("ISO Format"=→"ISO Format 3":T11, "DateTime.ISO8601 out"=→"DateTime.ISO8601 out 6":refnum<class "DateTime.ISO8601.lvclass">)  [unwired: 9 in]
      n28 = call <vilib>:"Write ISO Format.vi"("ISO Format"="ISO Format 2", "DateTime.ISO8601 in"="DateTime.ISO8601 in 5") -> ("DateTime.ISO8601 out"=→"DateTime.ISO8601 out 5":refnum<class "DateTime.ISO8601.lvclass">)  [unwired: 9 in]
      n29 = call <vilib>:"Read Support RFC3339.vi"("DateTime.ISO8601 in"="DateTime.ISO8601 in 4") -> ("Support RFC3339"=→"Support RFC3339":bool, "DateTime.ISO8601 out"=→"DateTime.ISO8601 out 4":refnum<class "DateTime.ISO8601.lvclass">)  [unwired: 9 in]
      n30 = call <vilib>:"Write Support RFC3339.vi"("Support RFC3339 (T)"="Support RFC3339 (T)", "DateTime.ISO8601 in"="DateTime.ISO8601 in 3") -> ("DateTime.ISO8601 out"=→"DateTime.ISO8601 out 3":refnum<class "DateTime.ISO8601.lvclass">)  [unwired: 9 in]
      n31 = call <vilib>:"YearToFirstDayW01.vi"("year"="year 2") -> ("First Day of W01"=→"First Day of W01":timestamp)  [unwired: 10 in]
      n32 = call <vilib>:"Adjust for DST.vi"("Adjust for DST? (T)"="Adjust for DST? (T)", "Timestamp"="Timestamp 8") -> ("Adjusted Timestamp"=→"Adjusted Timestamp":timestamp)  [unwired: 9 in]
      n33 = call <vilib>:"Timestamp to String.vi"("UTC? (F)"="UTC? (F) 9", "Timestamp (now)"="Timestamp (now) 8", "DateTimeFormatter in"="DateTimeFormatter in 4") -> ("Not a Timestamp?"=→"Not a Timestamp? 8":bool, "DateTime String"=→"DateTime String 4":string, "DateTimeFormatter out"=→"DateTimeFormatter out 4":refnum<class "DateTimeFormatter.lvclass">)  [unwired: 6 in]
      n34 = call <vilib>:"Timestamp from String.vi"("DateTime String"="DateTime String 3", "DateTimeFormatter in"="DateTimeFormatter in 3") -> ("Not a Timestamp?"=→"Not a Timestamp? 7":bool, "Timestamp"=→"Timestamp 7":timestamp, "DateTimeFormatter out"=→"DateTimeFormatter out 3":refnum<class "DateTimeFormatter.lvclass">)  [unwired: 7 in]
      n35 = call-dynamic "getOffsetToTAI.vi"("Epoch Time"="Epoch Time 3", "Epoch.GPS"="Epoch.GPS") -> ("Offset to TAI"=→"Offset to TAI 2":i64)  [unwired: 9 in]
      n36 = call-dynamic "getOffsetToUTC.vi"("Epoch (GPS)"="Epoch (GPS) 2") -> ("Offset to UTC"=→"Offset to UTC 4":i64)  [unwired: 10 in]
      n37 = call-dynamic "toTimestamp.vi"("Use TAI Offset?"="Use TAI Offset? 4", "Fractional Second"="Fractional Second 12", "GPS Time (s)"="GPS Time (s)", "Epoch (GPS)"="Epoch (GPS)") -> ("Not a Timestamp?"=→"Not a Timestamp? 6":bool, "Timestamp"=→"Timestamp 5":timestamp, "Epoch out"=→"Epoch out 11":refnum<class "Epoch.GPS.lvclass">)  [unwired: 5 in]
      n38 = call-dynamic "getOffsetToUTC.vi"("Epoch"="Epoch 4") -> ("Offset to UTC"=→"Offset to UTC 3":i64)  [unwired: 10 in]
      n39 = call-dynamic "getOffsetToTAI.vi"("Epoch Time"="Epoch Time 2", "Epoch"="Epoch 3") -> ("Offset to TAI"=→"Offset to TAI":i64)  [unwired: 9 in]
      n40 = call <vilib>:"timestampOffset.vi"("Reference Time"="Reference Time") -> ("Timestamp Offset"=→"Timestamp Offset":i64)  [unwired: 10 in]
      n41 = call-dynamic "toTimestamp.vi"("Use TAI Offset?"="Use TAI Offset? 3", "Fractional Second"="Fractional Second 11", "Epoch Time (s)"="Epoch Time (s) 3", "Epoch (Local)"="Epoch (Local) 2") -> ("Not a Timestamp?"=→"Not a Timestamp? 5":bool, "Timestamp"=→"Timestamp 4":timestamp, "Epoch (out)"=→"Epoch (out)":refnum<class "Epoch.lvclass">)  [unwired: 5 in]
      n42 = call <vilib>:"toDateTimeString.vi"("DateTimeFormatter (ISO8601)"="DateTimeFormatter (ISO8601)", "UTC? (F)"="UTC? (F) 7", "Fractional Second"="Fractional Second 10", "Epoch Time (s)"="Epoch Time (s) 2", "Epoch"="Epoch 2") -> ("Not a Timestamp?"=→"Not a Timestamp? 4":bool, "DateTime string"=→"DateTime string":string, "Epoch out"=→"Epoch out 10":refnum<class "Epoch.lvclass">)  [unwired: 4 in]
      n43 = call <vilib>:"leapSeconds LUT.vi"() -> ("Leap Seconds"=→"Leap Seconds 2":i64[], "UTC Time"=→"UTC Time":i64[])  [unwired: 10 in]
      n44 = call <vilib>:"getLeapSecondCount.vi"("UTC Epoch Time"="UTC Epoch Time") -> ("Leap Seconds"=→"Leap Seconds":i64)  [unwired: 10 in]
      n45 = call <vilib>:"mergeFractionalSeconds.vi"("Fractional Second"="Fractional Second 9", "(Integer) Time (s)"="(Integer) Time (s) 6", "Epoch in"="Epoch in 6") -> ("(Float) Time (s)"=→"(Float) Time (s) 2":dbl, "Epoch out"=→"Epoch out 9":refnum<class "Epoch.lvclass">)  [unwired: 7 in]
      n46 = call <vilib>:"mergeFractionalSeconds[ms].vi"("Fractional Second"="Fractional Second 8", "(Integer) Time (s)"="(Integer) Time (s) 5", "Epoch in"="Epoch in 5") -> ("(Integer) Time (ms)"=→"(Integer) Time (ms) 2":i64, "Epoch out"=→"Epoch out 8":refnum<class "Epoch.lvclass">)  [unwired: 7 in]
      n47 = call <vilib>:"mergeFractionalSeconds[us].vi"("Fractional Second"="Fractional Second 7", "(Integer) Time (s)"="(Integer) Time (s) 4", "Epoch in"="Epoch in 4") -> ("(Integer) Time (us)"=→"(Integer) Time (us) 2":i64, "Epoch out"=→"Epoch out 7":refnum<class "Epoch.lvclass">)  [unwired: 7 in]
      n48 = call <vilib>:"splitFractionalSeconds.vi"("(Float) Time (s)"="(Float) Time (s)", "Epoch in"="Epoch in 3") -> ("Fractional Second"=→"Fractional Second 6":dbl, "(Integer) Time (s)"=→"(Integer) Time (s) 3":i64, "Epoch out"=→"Epoch out 6":refnum<class "Epoch.lvclass">)  [unwired: 7 in]
      n49 = call <vilib>:"splitFractionalSeconds[ms].vi"("(Integer) Time (ms)"="(Integer) Time (ms)", "Epoch in"="Epoch in 2") -> ("Fractional Second"=→"Fractional Second 5":dbl, "(Integer) Time (s)"=→"(Integer) Time (s) 2":i64, "Epoch out"=→"Epoch out 5":refnum<class "Epoch.lvclass">)  [unwired: 7 in]
      n50 = call <vilib>:"splitFractionalSeconds[us].vi"("(Integer) Time (us)"="(Integer) Time (us)", "Epoch in"="Epoch in") -> ("Fractional Second"=→"Fractional Second 4":dbl, "(Integer) Time (s)"=→"(Integer) Time (s)":i64, "Epoch out"=→"Epoch out 4":refnum<class "Epoch.lvclass">)  [unwired: 7 in]
      n51 = call-dynamic "getOffsetToUTC.vi"("Epoch (UNIX)"="Epoch (UNIX)") -> ("Offset to UTC"=→"Offset to UTC 2":i64)  [unwired: 10 in]
      n52 = call-dynamic "toTimestamp.vi"("Use TAI Offset?"="Use TAI Offset? 2", "Fractional Second"="Fractional Second 3", "Unix Time (s)"="Unix Time (s)", "Epoch (Unix)"="Epoch (Unix)") -> ("Not a Timestamp?"=→"Not a Timestamp? 3":bool, "Timestamp"=→"Timestamp 3":timestamp, "Epoch out"=→"Epoch out 3":refnum<class "Epoch.UNIX.lvclass">)  [unwired: 5 in]
      n53 = call-dynamic "getOffsetToUTC.vi"("Epoch"="Epoch") -> ("Offset to UTC"=→"Offset to UTC":i64)  [unwired: 10 in]
      n54 = call-dynamic "toTimestamp.vi"("Use TAI Offset?"="Use TAI Offset?", "Fractional Second"="Fractional Second 2", "UTC Time (s)"="UTC Time (s)", "Epoch (UTC)"="Epoch (UTC) 2") -> ("Not a Timestamp?"=→"Not a Timestamp? 2":bool, "Timestamp"=→"Timestamp 2":timestamp, "Epoch out"=→"Epoch out 2":refnum<class "Epoch.UTC.lvclass">)  [unwired: 5 in]
      n55 = call <vilib>:"Error Cluster From Error Code.vi"("is warning? (False)"="is warning? (False)", "show call chain? (False)"="show call chain? (False)", "error in (no error)"="error in (no error) 33", "error message (\"\")"="error message (\"\")", "error code (0)"="error code (0)") -> ("error out"=→"error out 52":errorcluster)  [unwired: 4 in]
      n56 = call <vilib>:"Get Epoch Time.vi"("Timestamp (now)"="Timestamp (now) 6", "Epoch (Local)"="Epoch (Local)") -> ("Fractional Second"=→"Fractional Second":dbl, "Epoch Time (s)"=→"Epoch Time (s)":i64, "Epoch out"=→"Epoch out":refnum<class "Epoch.lvclass">)  [unwired: 7 in]
      n57 = call <vilib>:"Get File Extension.vi"("error in (no error)"="error in (no error) 32", "file"="file") -> ("error out"=→"error out 51":errorcluster, "filename without extension"=→"filename without extension":string, "lowercase file extension"=→"lowercase file extension":string, "dup file"=→"dup file":path, "unmodified file extension"=→"unmodified file extension":string)  [unwired: 5 in]
      n58 = call <vilib>:"Get Local UTC Offset.vi"("UTC? (F)"="UTC? (F) 6") -> ("UTC Offset String"=→"UTC Offset String 2":string, "UTC Offset"=→"UTC Offset 2":T1)  [unwired: 9 in]
      n59 = call <vilib>:"Get LV Class Name.vi"("error in (no error)"="error in (no error) 31", "object"="object") -> ("error out"=→"error out 50":errorcluster, "class name"=→"class name":string)  [unwired: 8 in]
      n60 = call <vilib>:"GregorianCal_MonthLengths.vi"("Year (0: this year)"="Year (0: this year) 2") -> ("Month Lengths"=→"Month Lengths":i32[])  [unwired: 10 in]
      n61 = call <vilib>:"ISO8601 DateString to Timestamp.vi"("Adjust for Local DST? (T)"="Adjust for Local DST? (T)", "Strict ISO? (T)"="Strict ISO? (T)", "ISO8601 Date String"="ISO8601 Date String") -> ("valid?"=→"valid?":bool, "ISO Format"=→"ISO Format":T11, "Timestamp"=→"Timestamp":timestamp)  [unwired: 6 in]
      n62 = call <vilib>:"create.vi"("error in"="error in 19", "Key"="Key", "Upload ID"="Upload ID") -> ("error out"=→"error out 49":errorcluster, "Nominal Client MultiPart Upload"=→"Nominal Client MultiPart Upload":refnum<class "Multipart Upload.lvclass">)  [unwired: 7 in]
      n63 = call <vilib>:"destroy.vi"("error in"="error in 18", "MultiPart Upload"="MultiPart Upload") -> ("error out"=→"error out 48":errorcluster)  [unwired: 9 in]
      n64 = call <vilib>:"upload.abort_multipart_upload.vi"("error in"="error in 17", "Multipart Upload"="Multipart Upload 4") -> ("error out"=→"error out 47":errorcluster)  [unwired: 9 in]
      n65 = call <vilib>:"upload.complete_multipart_upload.vi"("error in"="error in 16", "Multipart Upload in"="Multipart Upload in 3") -> ("error out"=→"error out 46":errorcluster, "S3 Path to File"=→"S3 Path to File":string)  [unwired: 8 in]
      n66 = call <vilib>:"upload.initiate_multipart_upload.vi"("error in"="error in 15", "File Path"="File Path", "Nominal Client in"="Nominal Client in") -> ("error out"=→"error out 45":errorcluster, "Multipart Upload"=→"Multipart Upload 3":refnum<class "Multipart Upload.lvclass">, "Nominal Client out"=→"Nominal Client out":refnum<class "Nominal Client.lvclass">)  [unwired: 6 in]
      n67 = call <vilib>:"upload.list_parts.vi"("error in"="error in 14", "Multipart Upload"="Multipart Upload 2") -> ("error out"=→"error out 44":errorcluster, "Multipart Upload out"=→"Multipart Upload out 4":refnum<class "Multipart Upload.lvclass">)  [unwired: 8 in]
      n68 = call <vilib>:"upload.part_core.vi"("error in"="error in 13", "Body"="Body", "Full Path"="Full Path", "REST Client"="REST Client") -> ("error out"=→"error out 43":errorcluster, "Response"=→"Response":string)  [unwired: 6 in]
      n69 = call <vilib>:"upload.sign_part.vi"("Part Number"="Part Number 2", "error in"="error in 12", "Multipart Upload in"="Multipart Upload in 2") -> ("error out"=→"error out 42":errorcluster, "Multipart Upload out"=→"Multipart Upload out 3":refnum<class "Multipart Upload.lvclass">)  [unwired: 7 in]
      n70 = call <vilib>:"upload.start_part_upload.vi"("Part Number"="Part Number", "error in"="error in 11", "File Part Binary"="File Part Binary", "Multipart Upload"="Multipart Upload") -> ("error out"=→"error out 41":errorcluster, "Multipart Upload out"=→"Multipart Upload out 2":refnum<class "Multipart Upload.lvclass">)  [unwired: 6 in]
      n71 = call <vilib>:"wait_to_finish_uploading.vi"("error in"="error in 10", "Multipart Upload in"="Multipart Upload in") -> ("error out"=→"error out 40":errorcluster, "Multipart Upload out"=→"Multipart Upload out":refnum<class "Multipart Upload.lvclass">)  [unwired: 8 in]
      n72 = call <vilib>:"All Palette VIs.vi"() -> ()  [unwired: 12 in]
      n73 = call <vilib>:"Get LabVIEW Class Default Palette Information.vi"("error in (no error)"="error in (no error) 30", "variant"="variant") -> ("error out"=→"error out 39":errorcluster, "default palette path"=→"default palette path":path)  [unwired: 8 in]
      n74 = call <vilib>:"Can File be in LLB.vi"("error in (no error)"="error in (no error) 29", "path"="path 9") -> ("error out"=→"error out 38":errorcluster, "Can be in LLB?"=→"Can be in LLB? 2":bool)  [unwired: 8 in]
      n75 = call <vilib>:"Get File Type.vi"("error in (no error)"="error in (no error) 28", "path"="path 8") -> ("error out"=→"error out 37":errorcluster, "is template?"=→"is template? 2":bool, "file type"=→"file type 6":T9)  [unwired: 7 in]
      n76 = call <vilib>:"Get File Type Icon Image.vi"("error in (no error)"="error in (no error) 27", "path"="path 7") -> ("error out"=→"error out 36":errorcluster, "image data"=→"image data 2":T10)  [unwired: 8 in]
      n77 = call <vilib>:"Is File a LabVIEW document.vi"("error in (no error)"="error in (no error) 26", "path"="path 6") -> ("error out"=→"error out 35":errorcluster, "Is LabVIEW document?"=→"Is LabVIEW document? 2":bool)  [unwired: 8 in]
      n78 = call <vilib>:"Is File a type of library.vi"("error in (no error)"="error in (no error) 25", "path"="path 5") -> ("error out"=→"error out 34":errorcluster, "Is library type?"=→"Is library type? 2":bool)  [unwired: 8 in]
      n79 = call <vilib>:"Is File VI.vi"("error in (no error)"="error in (no error) 24", "path"="path 4") -> ("error out"=→"error out 33":errorcluster, "Is Class Private Data Control?"=→"Is Class Private Data Control?":bool, "Is VI?"=→"Is VI? 2":bool)  [unwired: 7 in]
      n80 = call <vilib>:"Is File an LLB.vi"("error in (no error)"="error in (no error) 23", "path"="path 3") -> ("error out"=→"error out 32":errorcluster, "Is LLB?"=→"Is LLB?":bool)  [unwired: 8 in]
      n81 = call <vilib>:"Convert filetype to Is VI.vi"("file type"="file type 5") -> ("Is VI?"=→"Is VI?":bool)  [unwired: 4 in]
      n82 = call <vilib>:"Convert filetype to Icon Image.vi"("error in (no error)"="error in (no error) 22", "is template?"="is template?", "file type"="file type 4") -> ("error out"=→"error out 31":errorcluster, "image data"=→"image data":T10)  [unwired: 7 in]
      n83 = call <vilib>:"Convert filetype to Can be in LLB.vi"("file type"="file type 3") -> ("Can be in LLB?"=→"Can be in LLB?":bool)  [unwired: 4 in]
      n84 = call <vilib>:"Convert filetype to Is library type.vi"("file type"="file type 2") -> ("Is library type?"=→"Is library type?":bool)  [unwired: 4 in]
      n85 = call <vilib>:"Convert filetype to Is LabVIEW document.vi"("file type"="file type") -> ("Is LabVIEW document?"=→"Is LabVIEW document?":bool)  [unwired: 4 in]
      n86 = call <vilib>:"Enable Caching.vi"("error in (no error)"="error in (no error) 21", "Enable"="Enable") -> ("error out"=→"error out 30":errorcluster)  [unwired: 3 in]
      n87 = call <vilib>:"Get Exported File List.vi"("error in (no error)"="error in (no error) 20", "packed library path"="packed library path 5") -> ("error out"=→"error out 29":errorcluster, "paths"=→"paths":path[], "qualified names"=→"qualified names":string[])  [unwired: 7 in]
      n88 = call <vilib>:"Get Exported File Path.vi"("error in (no error)"="error in (no error) 19", "qualified name"="qualified name", "packed library path"="packed library path 4") -> ("error out"=→"error out 28":errorcluster, "path"=→"path 2":path)  [unwired: 7 in]
      n89 = call <vilib>:"Get Guid String.vi"("error in (no error)"="error in (no error) 18", "packed library path"="packed library path 3") -> ("error out"=→"error out 27":errorcluster, "guid"=→"guid":string)
      n90 = call <vilib>:"Get Source Project Path.vi"("error in (no error)"="error in (no error) 17", "packed library path"="packed library path 2") -> ("error out"=→"error out 26":errorcluster, "source project path"=→"source project path":path)
      n91 = call <vilib>:"Packed Library Path.vi"("error in (no error)"="error in (no error) 16", "vi reference"="vi reference") -> ("error out"=→"error out 25":errorcluster, "packed library path"=→"packed library path":path, "vi reference out"=→"vi reference out":refnum<vi>)  [unwired: 1 in]
      n92 = call <vilib>:"Get Header By Name.vi"("error in (no error)"="error in (no error) 15", "Name"="Name", "Response Headers in"="Response Headers in 2") -> ("error out"=→"error out 22":errorcluster, "Found?"=→"Found?":bool, "Value"=→"Value":string, "Response Headers out"=→"Response Headers out 2":refnum<class "Response Headers.lvclass">)  [unwired: 5 in]
      n93 = call <vilib>:"Get All Headers.vi"("error in (no error)"="error in (no error) 14", "Response Headers in"="Response Headers in") -> ("error out"=→"error out 21":errorcluster, "Values"=→"Values":string[], "Names"=→"Names":string[], "Response Headers out"=→"Response Headers out":refnum<class "Response Headers.lvclass">)  [unwired: 6 in]
      n94 = call <vilib>:"Create REST Client.vi"("Default Headers ([JSON])"="Default Headers ([JSON])", "REST Client in"="REST Client in 9", "Verify Server(true)"="Verify Server(true)", "Cookie File"="Cookie File", "error in (no error)"="error in (no error) 13", "Authentication"="Authentication", "Escape URLs (true)"="Escape URLs (true)", "Base URL"="Base URL") -> ("error out"=→"error out 20":errorcluster, "REST Client out"=→"REST Client out 8":refnum<class "REST Client.lvclass">)  [unwired: 2 in]
      n95 = call-dynamic "HTTP HEAD.vi"("request specific headers"="request specific headers 7", "timeout (0 = Use Default)"="timeout (0 = Use Default) 7", "error in (no error)"="error in (no error) 12", "Path"="Path 7", "REST Client in"="REST Client in 8") -> ("error out"=→"error out 19":errorcluster, "Response body"=→"Response body 7":string, "Response Headers"=→"Response Headers 7":refnum<class "Response Headers.lvclass">, "REST Client out"=→"REST Client out 7":refnum<class "REST Client.lvclass">, "Status String"=→"Status String 7":string, "Status Code"=→"Status Code 7":u16)  [unwired: 1 in]
      n96 = call-dynamic "HTTP GET.vi"("request specific headers"="request specific headers 6", "timeout (0 = Use Default)"="timeout (0 = Use Default) 6", "error in (no error)"="error in (no error) 11", "Path"="Path 6", "REST Client in"="REST Client in 7") -> ("error out"=→"error out 18":errorcluster, "Response body"=→"Response body 6":string, "Response Headers"=→"Response Headers 6":refnum<class "Response Headers.lvclass">, "REST Client out"=→"REST Client out 6":refnum<class "REST Client.lvclass">, "Status String"=→"Status String 6":string, "Status Code"=→"Status Code 6":u16)  [unwired: 1 in]
      n97 = call-dynamic "HTTP PUT.vi"("request specific headers"="request specific headers 5", "timeout (0 = Use Default)"="timeout (0 = Use Default) 5", "error in (no error)"="error in (no error) 10", "Request body"="Request body 3", "Path"="Path 5", "REST Client in"="REST Client in 6") -> ("error out"=→"error out 17":errorcluster, "Response body"=→"Response body 5":string, "Response Headers"=→"Response Headers 5":refnum<class "Response Headers.lvclass">, "REST Client out"=→"REST Client out 5":refnum<class "REST Client.lvclass">, "Status String"=→"Status String 5":string, "Status Code"=→"Status Code 5":u16)
      n98 = call-dynamic "HTTP POST.vi"("request specific headers"="request specific headers 4", "timeout (0 = Use Default)"="timeout (0 = Use Default) 4", "error in (no error)"="error in (no error) 9", "Request body"="Request body 2", "Path"="Path 4", "REST Client in"="REST Client in 5") -> ("error out"=→"error out 16":errorcluster, "Response body"=→"Response body 4":string, "Response Headers"=→"Response Headers 4":refnum<class "Response Headers.lvclass">, "REST Client out"=→"REST Client out 4":refnum<class "REST Client.lvclass">, "Status String"=→"Status String 4":string, "Status Code"=→"Status Code 4":u16)
      n99 = call-dynamic "HTTP POST Multipart.vi"("request specific headers"="request specific headers 3", "timeout (0 = Use Default)"="timeout (0 = Use Default) 3", "error in (no error)"="error in (no error) 8", "Multipart Post data"="Multipart Post data", "Path"="Path 3", "REST Client in"="REST Client in 4") -> ("error out"=→"error out 15":errorcluster, "Response body"=→"Response body 3":string, "Response Headers"=→"Response Headers 3":refnum<class "Response Headers.lvclass">, "REST Client out"=→"REST Client out 3":refnum<class "REST Client.lvclass">, "Status String"=→"Status String 3":string, "Status Code"=→"Status Code 3":u16)
      n100 = call-dynamic "HTTP DELETE.vi"("request specific headers"="request specific headers 2", "timeout (0 = Use Default)"="timeout (0 = Use Default) 2", "error in (no error)"="error in (no error) 7", "Path"="Path 2", "REST Client in"="REST Client in 3") -> ("error out"=→"error out 14":errorcluster, "Response body"=→"Response body 2":string, "Response Headers"=→"Response Headers 2":refnum<class "Response Headers.lvclass">, "REST Client out"=→"REST Client out 2":refnum<class "REST Client.lvclass">, "Status String"=→"Status String 2":string, "Status Code"=→"Status Code 2":u16)  [unwired: 1 in]
      n101 = call-dynamic "HTTP PATCH.vi"("request specific headers"="request specific headers", "timeout (0 = Use Default)"="timeout (0 = Use Default)", "error in (no error)"="error in (no error) 6", "Request body"="Request body", "Path"="Path", "REST Client in"="REST Client in 2") -> ("error out"=→"error out 13":errorcluster, "Response body"=→"Response body":string, "Response Headers"=→"Response Headers":refnum<class "Response Headers.lvclass">, "REST Client out"=→"REST Client out":refnum<class "REST Client.lvclass">, "Status String"=→"Status String":string, "Status Code"=→"Status Code":u16)
      n102 = call-dynamic "Destroy REST Client.vi"("error in (no error)"="error in (no error) 5", "REST Client in"="REST Client in") -> ("error out"=→"error out 12":errorcluster)  [unwired: 9 in]
      n103 = call <vilib>:"create.vi"("Run Data"="Run Data") -> ("Run"=→"Run":refnum<class "Run.lvclass">)
      n104 = call <vilib>:"Timestamp to ISO8601 Date.vi"("UTC? (F)"="UTC? (F) 5", "Timestamp (now)"="Timestamp (now) 5") -> ("ISO8601 Calendar Month"=→"ISO8601 Calendar Month":string, "ISO8601 Date"=→"ISO8601 Date":string)  [unwired: 8 in]
      n105 = call <vilib>:"Timestamp to ISO8601 Day.vi"("UTC? (F)"="UTC? (F) 4", "Timestamp (now)"="Timestamp (now) 4") -> ("Day of Year"=→"Day of Year":i32, "ISO Weekday"=→"ISO Weekday":i32, "ISO Day"=→"ISO Day":T4)  [unwired: 7 in]
      n106 = call <vilib>:"Timestamp to ISO8601 UTC DateTime.vi"("UTC? (F)"="UTC? (F) 3", "Timestamp (now)"="Timestamp (now) 3") -> ("ISO8601 UTC DateTime"=→"ISO8601 UTC DateTime":string)  [unwired: 9 in]
      n107 = call <vilib>:"Timestamp to ISO8601 Week.vi"("UTC? (F)"="UTC? (F) 2", "Timestamp (now)"="Timestamp (now) 2") -> ("ISO8601 Ordinal Date"=→"ISO8601 Ordinal Date":string, "ISO8601 Weekday"=→"ISO8601 Weekday":string, "ISO8601 Week"=→"ISO8601 Week":string)  [unwired: 7 in]
      n108 = call <vilib>:"Timestamp to ISO8601 Year.vi"("UTC? (F)"="UTC? (F)", "Timestamp (now)"="Timestamp (now)") -> ("is Leap Year?"=→"is Leap Year?":bool, "year"=→"year":i32)  [unwired: 8 in]
      n109 = call <vilib>:"build.ts.vi"() -> ("timestampMetadata out"=→"timestampMetadata out 5":refnum<class "timestampMetadata.lvclass">)  [unwired: 11 in]
      n110 = call-dynamic "json.generate_object.vi"("error in"="error in 7", "timestampMetadata in"="timestampMetadata in 3") -> ("error out"=→"error out 11":errorcluster, "JSON Object"=→"JSON Object 4":string, "timestampMetadata out"=→"timestampMetadata out 4":refnum<class "timestampMetadata.lvclass">)  [unwired: 7 in]
      n111 = call <vilib>:"json.insert.vi"("error in"="error in 6", "Object Name"="Object Name", "JSON in"="JSON in 2", "timestampMetadata in"="timestampMetadata in 2") -> ("error out"=→"error out 10":errorcluster, "JSON out"=→"JSON out 2":string, "timestampMetadata out"=→"timestampMetadata out 3":refnum<class "timestampMetadata.lvclass">)  [unwired: 5 in]
      n112 = call <vilib>:"json.replace.vi"("error in"="error in 5", "Object To Update"="Object To Update", "JSON in"="JSON in", "timestampMetadata in"="timestampMetadata in") -> ("error out"=→"error out 9":errorcluster, "JSON out"=→"JSON out":string, "timestampMetadata out"=→"timestampMetadata out 2":refnum<class "timestampMetadata.lvclass">)  [unwired: 5 in]
      n113 = call <vilib>:"Trim Whitespace One-Sided.vi"("string"="string 2", "reverse?"="reverse?", "enable?"="enable?") -> ("trimmed string"=→"trimmed string 2":string)
      n114 = call <vilib>:"Trim Whitespace.vi"("string"="string", "location (both)"="location (both)") -> ("trimmed string"=→"trimmed string":string)
      n115 = call <vilib>:"build.epoch.vi"("Time Unit"="Time Unit 2", "Time Series Name"="Time Series Name 3") -> ("ts.epochOfTimeUnit out"=→"ts.epochOfTimeUnit out 2":refnum<class "ts.epochOfTimeUnit.lvclass">)  [unwired: 9 in]
      n116 = call-dynamic "json.generate_object.vi"("error in"="error in 4", "ts.epochOfTimeUnit in"="ts.epochOfTimeUnit in") -> ("error out"=→"error out 8":errorcluster, "JSON Object"=→"JSON Object 3":string, "ts.epochOfTimeUnit out"=→"ts.epochOfTimeUnit out":refnum<class "ts.epochOfTimeUnit.lvclass">)  [unwired: 7 in]
      n117 = call <vilib>:"build.iso8601.vi"("Time Series Name"="Time Series Name 2") -> ("ts.iso8601 out"=→"ts.iso8601 out 2":refnum<class "ts.iso8601.lvclass">)  [unwired: 10 in]
      n118 = call-dynamic "json.generate_object.vi"("error in"="error in 3", "ts.iso8601 in"="ts.iso8601 in") -> ("error out"=→"error out 7":errorcluster, "JSON Object"=→"JSON Object 2":string, "ts.iso8601 out"=→"ts.iso8601 out":refnum<class "ts.iso8601.lvclass">)  [unwired: 7 in]
      n119 = call <vilib>:"build.relative.vi"("Time Unit"="Time Unit", "Time Series Name"="Time Series Name") -> ("ts.relative out"=→"ts.relative out 2":refnum<class "ts.relative.lvclass">)  [unwired: 9 in]
      n120 = call-dynamic "json.generate_object.vi"("error in"="error in 2", "ts.relative in"="ts.relative in") -> ("error out"=→"error out 6":errorcluster, "JSON Object"=→"JSON Object":string, "ts.relative out"=→"ts.relative out":refnum<class "ts.relative.lvclass">)  [unwired: 7 in]
      n121 = call <vilib>:"UTC Offset to Seconds.vi"("UTC Offset String"="UTC Offset String") -> ("Valid?"=→"Valid?":bool, "Offset (s)"=→"Offset (s)":ext, "UTC Offset"=→"UTC Offset":T1, "UTC Offset?"=→"UTC Offset?":bool)  [unwired: 7 in]
      n122 = call <vilib>:"Write Delimited Spreadsheet (DBL).vi"("file path (dialog if empty)"="file path (dialog if empty) 5", "format (%.3f)"="format (%.3f) 2", "2D data"="2D data 4", "1D data"="1D data 4", "append to file? (new file:F)"="append to file? (new file:F) 5", "error in (no error)"="error in (no error) 4", "transpose? (no:F)"="transpose? (no:F) 4", "delimiter (\\t)"="delimiter (\\t) 4") -> ("new file path (Not A Path if cancelled)"=→"new file path (Not A Path if cancelled) 4":path, "error out"=→"error out 5":errorcluster)  [unwired: 6 in]
      n123 = call <vilib>:"Write Delimited Spreadsheet (I64).vi"("file path (dialog if empty)"="file path (dialog if empty) 4", "format (%d)"="format (%d)", "2D data"="2D data 3", "1D data"="1D data 3", "append to file? (new file:F)"="append to file? (new file:F) 4", "error in (no error)"="error in (no error) 3", "transpose? (no:F)"="transpose? (no:F) 3", "delimiter (\\t)"="delimiter (\\t) 3") -> ("new file path (Not A Path if cancelled)"=→"new file path (Not A Path if cancelled) 3":path, "error out"=→"error out 4":errorcluster)  [unwired: 6 in]
      n124 = call <vilib>:"Write Delimited Spreadsheet (string).vi"("file path (dialog if empty)"="file path (dialog if empty) 3", "format (%s)"="format (%s)", "2D data"="2D data 2", "1D data"="1D data 2", "append to file? (new file:F)"="append to file? (new file:F) 3", "error in (no error)"="error in (no error) 2", "transpose? (no:F)"="transpose? (no:F) 2", "delimiter (\\t)"="delimiter (\\t) 2") -> ("new file path (Not A Path if cancelled)"=→"new file path (Not A Path if cancelled) 2":path, "error out"=→"error out 3":errorcluster)  [unwired: 6 in]
      n125 = call-poly <vilib>:"Write Delimited Spreadsheet.vi"("file path (dialog if empty)"="file path (dialog if empty) 2", "format (%.3f)"="format (%.3f)", "2D data"="2D data", "1D data"="1D data", "append to file? (new file:F)"="append to file? (new file:F) 2", "error in (no error)"="error in (no error)", "transpose? (no:F)"="transpose? (no:F)", "delimiter (\\t)"="delimiter (\\t)") -> ("new file path (Not A Path if cancelled)"=→"new file path (Not A Path if cancelled)":path, "error out"=→"error out 2":errorcluster)  [unwired: 6 in]
      n126 = call <vilib>:"Write Spreadsheet String.vi"("prompt"="prompt", "error in"="error in", "append to file? (new file:F)"="append to file? (new file:F)", "spreadsheet string"="spreadsheet string", "file path (dialog if empty)"="file path (dialog if empty)") -> ("error out"=→"error out":errorcluster, "path"=→"path":path)  [unwired: 5 in]
      n127 = call-poly <vilib>:"timestamp.create.vi"() -> ("timestampMetadata out"=→"timestampMetadata out":refnum<class "timestampMetadata.lvclass">)  [unwired: 11 in]
    }
    frame Enabled {
    }
  }
